vi "BrowsePi.vi"() -> (1 "Code out":string, 2 "Success?":bool)   [LabVIEW 2019]
panel:
  in  "Save Button":bool
  in  "OK Button":bool
  in  "Cancel Button":bool
  in  "Code":string
  in  "Files":i32(listbox)=3
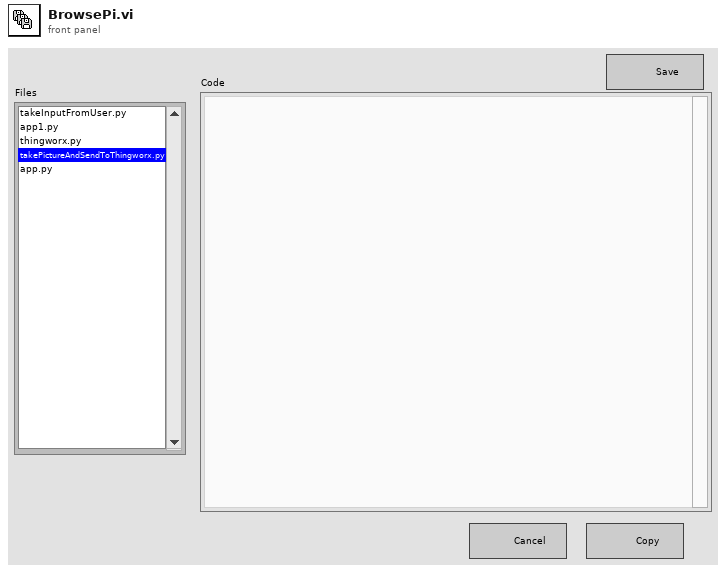
[diagram p1: front panel]
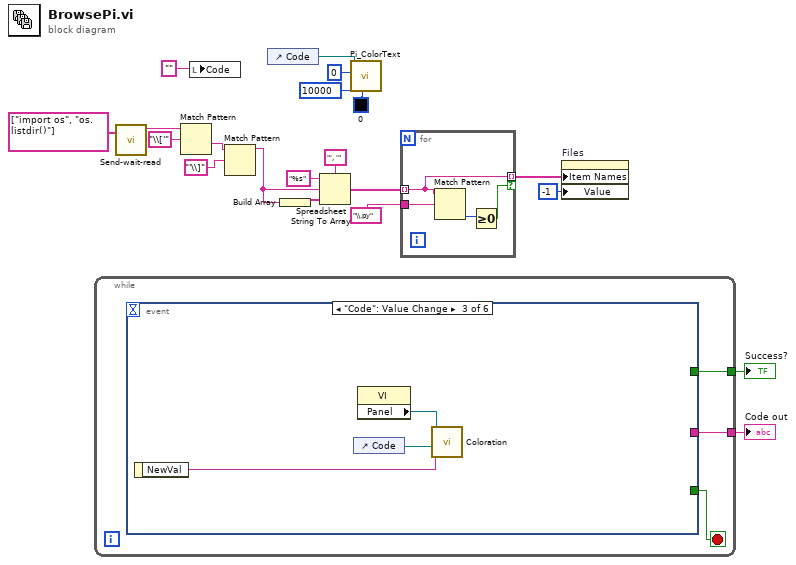
[diagram p0: block diagram]
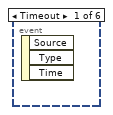
[diagram p2: hidden frame]
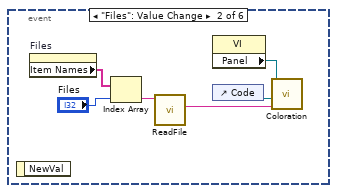
[diagram p3: hidden frame]
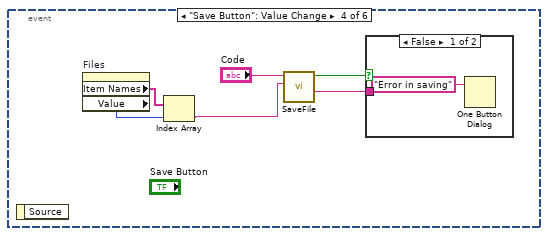
[diagram p4: hidden frame]
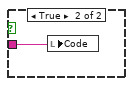
[diagram p5: hidden frame]
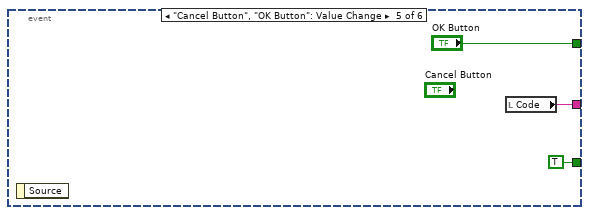
[diagram p6: hidden frame]
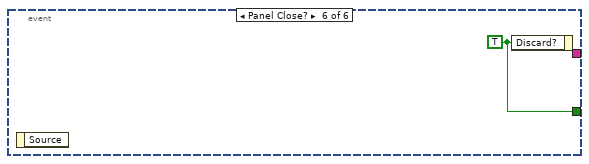
[diagram p7: hidden frame]
diagram:
  n1 = while {
    tunnel: [w22] -> w9
    tunnel: [w21] -> w7
    stop <- w23 stop-if-true
    n2 = event shown="[2] \"Code\": Value Change" {
      selector: _ -> [_ _ _ _ _ _]
      dyn-events: _ -> [_ _ _ _ _ _]
      timeout: _ -> [_ _ _ _ _ _]
      tunnel: [_ _ _ _ TRUE ("Discard?") w44] -> w23
      tunnel: [_ _ _ _ "OK Button" _] -> w22
      tunnel: [_ _ _ _ w41 _] -> w21
      event Timeout {
        n3 = event-data() -> ()  [unwired: 1 in, 3 out]
      }
      event "Files": Value Change {
        n4 = event-data() -> ()  [unwired: 1 in, 1 out]
        n5 = property on="Files" class="LstBox (strict)"() -> ("Item Names"=w28:string[])  [unwired: 2 in, 2 out]
        n6 = Index Array(array=w28, index="Files") -> (element=w27:string)
        n7 = call "ReadFile.vi"("String"=w27) -> ("file contents"=w26:string)  [unwired: 9 in, 1 out]
        n8 = property class="VI"() -> ("Panel"=w25:refnum<vi>)  [unwired: 2 in, 2 out]
        n9 = control-ref of="Code"() -> (w24:refnum<vi>)
        n10 = call "Coloration.vi"("String"=w26, "Code"=w24, "Front Panel"=w25) -> ()  [unwired: 9 in]
      }
      event "Code": Value Change {
        n11 = event-data() -> ("NewVal"=w30:string)  [unwired: 1 in]
        n12 = control-ref of="Code"() -> (w31:refnum<vi>)
        n13 = property class="VI"() -> ("Panel"=w32:refnum<vi>)  [unwired: 2 in, 2 out]
        n14 = call "Coloration.vi"("String"=w30, "Code"=w31, "Front Panel"=w32) -> ()  [unwired: 9 in]
      }
      event "Save Button": Value Change {
        n15 = event-data() -> ()  [unwired: 1 in, 1 out]
        n16 = property on="Files" class="LstBox (strict)"() -> ("Item Names"=w36:string[], "Value"=w35:i32)  [unwired: 2 in, 2 out]
        n17 = Index Array(array=w36, index=w35) -> (element=w34:string)
        n18 = call "SaveFile.vi"("Name"=w34, "Code"="Code") -> ("file contents"=w38:string, "Success?"=w37:bool)  [unwired: 8 in]
        n19 = case shown="False" w37 {
          tunnel: w38 -> [_ w40]
          frame False {
            n20 = One Button Dialog(message="Error in saving") -> ()  [unwired: 1 in, 1 out]
          }
          frame True {
            n21 = local write "Code"(w40) -> ()
          }
        }
      }
      event "Cancel Button", "OK Button": Value Change {
        n22 = event-data() -> ()  [unwired: 1 in, 1 out]
        n23 = local read "Code"() -> (w41:string)
      }
      event Panel Close? {
        w44 = TRUE ("Discard?")
        n24 = event-data() -> ()  [unwired: 1 in, 1 out]
        n25 = event-data("Discard?"=w44) -> ()  [unwired: 1 in, 1 out]
      }
    }
  }
  "Success?" <- w9
  "Code out" <- w7
  n26 = call "Send-wait-read.vi"("commands"=string[] ["import os", "os.listdir()"]) -> ("Last string"=w12:string)  [unwired: 9 in, 1 out]
  n27 = Match Pattern(string=w12, regular expression="\\['") -> (after substring=w19:string)  [unwired: 1 in, 3 out]
  n28 = local write "Code"("" ("Code")) -> ()
  n29 = Match Pattern(string=w19, regular expression="'\\]") -> (before substring=w16:string)  [unwired: 1 in, 3 out]
  n30 = control-ref of="Code"() -> (w1:refnum<vi>)
  n31 = Build Array(w16) -> (w15:string[])
  n32 = Spreadsheet String To Array(delimiter (Tab)="', '", format string="%s", spreadsheet string=w16, array type (2D Dbl)=w15) -> (array=w6:string[])
  n33 = call "Pi_ColorText.vi"("Color"=u32 0, "End"=10000, "Start"=0, "String in"=w1) -> ()  [unwired: 7 in, 1 out]
  n34 = for {
    tunnel: w6 -> [w46] mode=indexing
    tunnel: "\\.py" ("delimiter (Tab)") -> [w48]
    tunnel: [w46] -> w5 mode=indexing if=w45
    n35 = Match Pattern(string=w46, regular expression=w48) -> (offset past match=w47:i32)  [unwired: 1 in, 3 out]
    n36 = Greater Or Equal To 0?(x=w47) -> (x >= 0?=w45:bool)
  }
  n37 = property on="Files" class="LstBox (strict)"("Item Names"=w5, "Value"=-1 ("Files")) -> ()  [unwired: 2 in, 2 out]
